vi "aft_Fill_In_Error_Info.vi"(7 "depth":i32=1, 8 "error in":errorcluster, 9 "extended error info":string, 10 "status code":i32) -> (0 "error out":errorcluster)   [LabVIEW 2017, in "NI_AdaptiveFilter.lvlib"]
doc: "Fill in error information."
uses:
  <vilib>/addons/Adaptive Filters/NI_AdaptiveFilter.lvlib
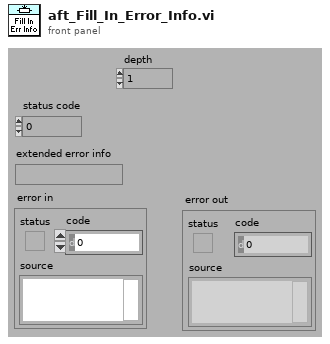
[diagram p1: front panel]
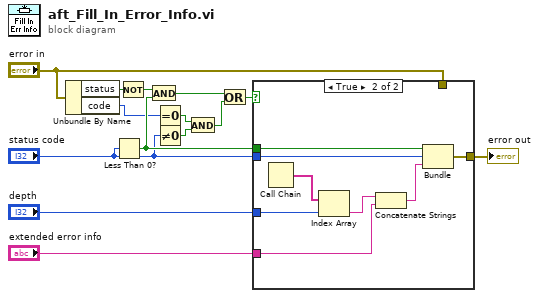
[diagram p0: block diagram]
diagram:
  n1 = Unbundle By Name("error in") -> ("status"=w6:bool, "code"=w11:i32)
  n2 = Less Than 0?(x="status code") -> (x < 0?=w12:bool)
  n3 = Not(x=w6) -> (.not. x?=w10:bool)
  n4 = And(x=w10, y=w12) -> (x .and. y?=w7:bool)
  n5 = Equal To 0?(x=w11) -> (x = 0?=w5:bool)
  n6 = Not Equal To 0?(x="status code") -> (x != 0?=w8:bool)
  n7 = And(x=w5, y=w8) -> (x .and. y?=w4:bool)
  n8 = Or(x=w7, y=w4) -> (x .or. y?=w3:bool)
  n9 = case shown="True" w3 {
    tunnel: [w15 w22] -> w13
    tunnel: "status code" -> [_ w21]
    tunnel: w12 -> [_ w20]
    tunnel: "error in" -> [w15 _]
    tunnel: "depth" -> [_ w17]
    tunnel: "extended error info" -> [_ w16]
    frame False {
    }
    frame True {
      n10 = Call Chain() -> (call chain=w19:string[])
      n11 = Index Array(array=w19, index=w17) -> (element=w18:string)
      n12 = Concatenate Strings(w18, w16) -> (w23:string)
      n13 = Bundle(w20, "status code"=w21, w23) -> (w22:cluster{bool, "status code":i32, string})  [unwired: 1 out]
    }
  }
  "error out" <- w13
